vi "set temperature program.vi"(8 "Detectors":T2, 11 "Serial Port":refnum<visa-resource-name>) -> (0 "Canceled":bool, 1 "run time":dbl format="%<%H:%M:%S%0u>t", 2 "delta x":dbl=0.05 format="%.5f", 3 "Serial Port":refnum<visa-resource-name>, 4 "data points":u8)   [LabVIEW 2012]
uses:
  detector.ctl
panel:
  in  "data rate":T1(ring)
  in  "Inj B Temp":u16=100 max=400 step=1
  in  "cancel":bool
  out "Message":string
  out "response":string[](array[string])
  in  "Ramps":T3(ring)
  in  "Oven Equilibrium time":sgl=10.0 min=0 max=650 step=0.01 format="%.2f"
  in  "Oven Temperature":T4={"initial temp"=0, "initial time"=0.0, "rate"=10.0, "final temp"=0, "final time"=0.0, "rate A"=0.0, "final temp A"=0, "final time A"=1.4013e-43, "rate B"=10.0, "final temp B"=0, "final time B"=0.0} {"initial temp" min=-80 max=450 step=1; "final temp B" min=-80 max=450 step=1; "initial time" min=0 max=650 step=0.01 format="%.2f"; "final time B" min=0 max=650 step=0.01 format="%.2f"; "final temp A" min=-80 max=450 step=1; "rate B" min=0 max=70 step=0.1 format="%.1f"; "final time A" min=0 max=650 step=0.01 format="%.2f"; "final temp" min=-80 max=450 step=1; "rate A" min=0 max=70 step=0.1 format="%.1f"; "final time" min=0 max=650 step=0.01 format="%.2f"; "rate" min=0 max=70 step=0.1 format="%.1f"}
  in  "done":bool
  out "Temperatures":cluster{sgl[], u16[]}[](graph)
  in  "Det B temp":u16=100 max=400 step=1
  in  "Det A temp":u16=100 max=450 step=1
  in  "Inj A Temp":u16=100 max=400 step=1
  # "°C"
  # "Decimal minutes"
  # "Temperatures"
  # "times in decimal minutes\ntemperatures in °C"
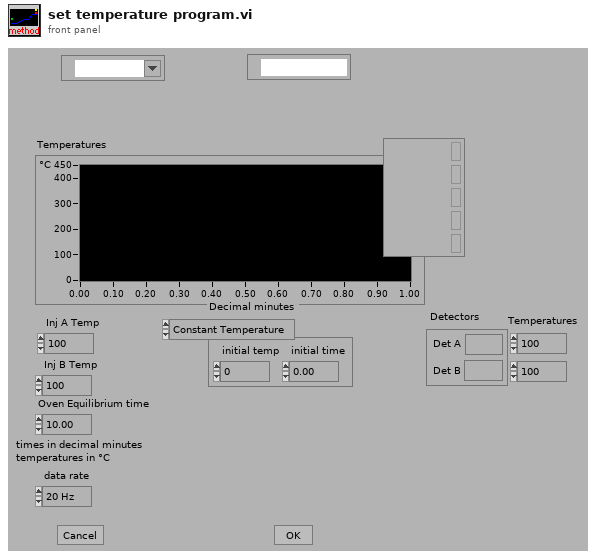
[diagram p1: front panel]
types:
  T1 = enum16{"20 Hz", "10 Hz", "5 Hz", "2.5 Hz", "1.25 Hz"}
  T2 = typedef "detector.ctl" = cluster{"Det A":string, "Det B":string}
  T3 = enum16{"Constant Temperature", "One Temperature Ramp", "Two Temperature Ramps", "Three Temperature Ramps"}
  T4 = cluster{"initial temp":i16, "initial time":sgl, "rate":sgl, "final temp":i16, "final time":sgl, "rate A":sgl, "final temp A":i16, "final time A":sgl, "rate B":sgl, "final temp B":i16, "final time B":sgl}
  T5 = cluster{"Version":sgl, "Initial Temp":sgl, "Oven On/Off":sgl, "Cryogenic  On/Off":sgl, "Oven Max":sgl, "Equib Time":sgl, "Initial Time":sgl, "Rate":dbl, "Final Temp":dbl, "Final Time":dbl, "Rate A":dbl, "Final Temp A":dbl, "Final Time A":dbl, "Rate B":dbl, "Final Temp B":dbl, "Final Time B":dbl, "Inj. A Temp":dbl, "Inj. A Temp On/Off":dbl, "Inj. B Temp":dbl, "Inj. B Temp On/Off":dbl, "Det. A Temp":dbl, "Det. A Temp On/Off":dbl, "Det. B Temp":dbl, "Det. B Temp On/Off":dbl, "Signal 1 Address":dbl, "Signal 1 Range":dbl, "Signal 1 Zero":dbl, "Signal 1 Zero On/Off":dbl, "Signal 1 Attn.":dbl, "Signal 1 Attn. On/Off":dbl, "Signal 2 Address":dbl, "Signal 2 Range":dbl, "Signal 2 Zero":dbl, "Signal 2 Zero On/Off":dbl, "Signal 2 Attn.":dbl, "Signal 2 Attn. On/Off":dbl, "Det. A On/Off":dbl, "Det. A Polarity":dbl, "Det. A Time":dbl, "Det. B On/Off":dbl, "Det. B Polarity":dbl, "Det. B Time":dbl, "Purge A On/Off":dbl, "Purge A On Time":dbl, "Purge A Off Time":dbl, "Purge B On/Off":dbl, "Purge B On Time":dbl, "Purge B Off Time":dbl}
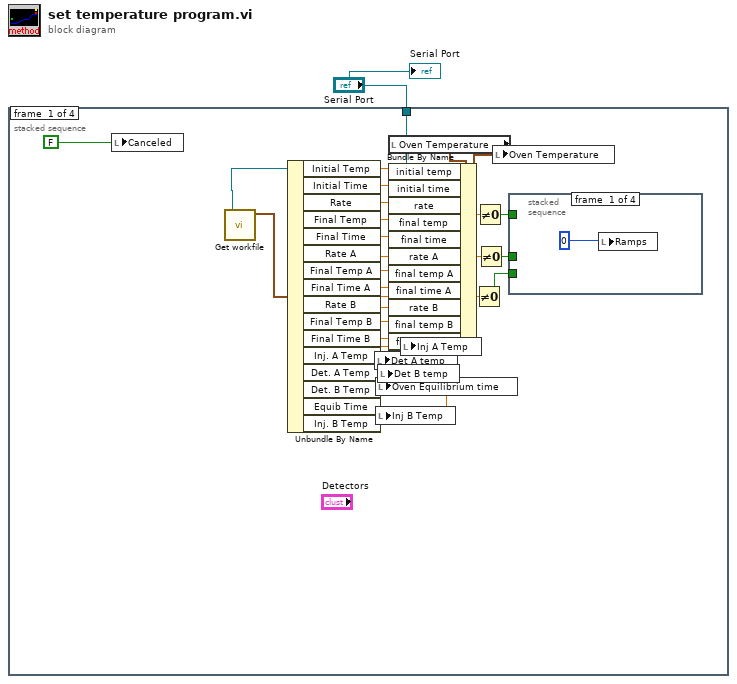
[diagram p0: block diagram]
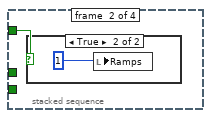
[diagram p2: hidden frame]
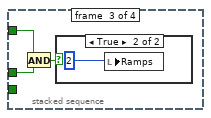
[diagram p4: hidden frame]
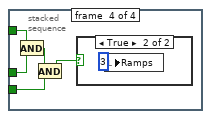
[diagram p6: hidden frame]
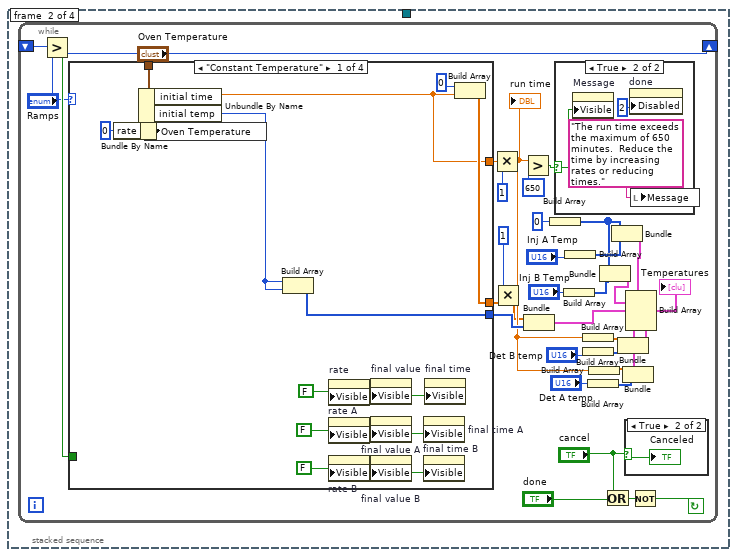
[diagram p8: hidden frame]
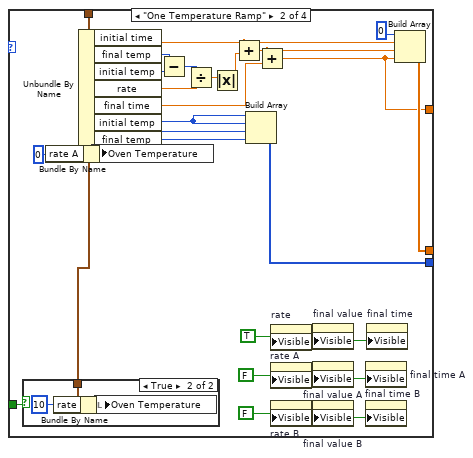
[diagram p10: hidden frame]
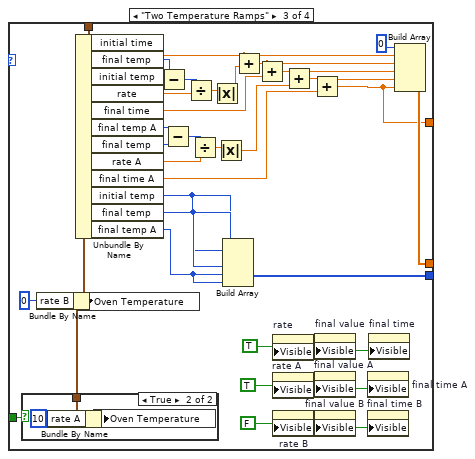
[diagram p12: hidden frame]
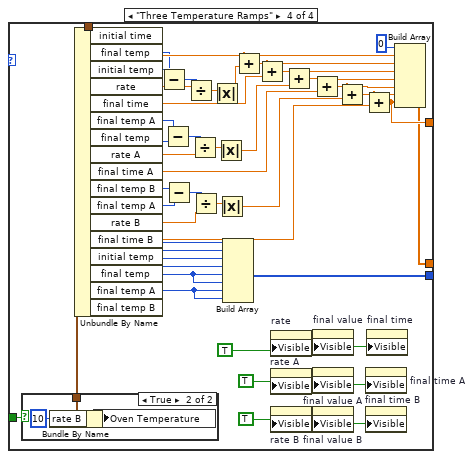
[diagram p14: hidden frame]
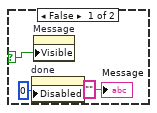
[diagram p16: hidden frame]
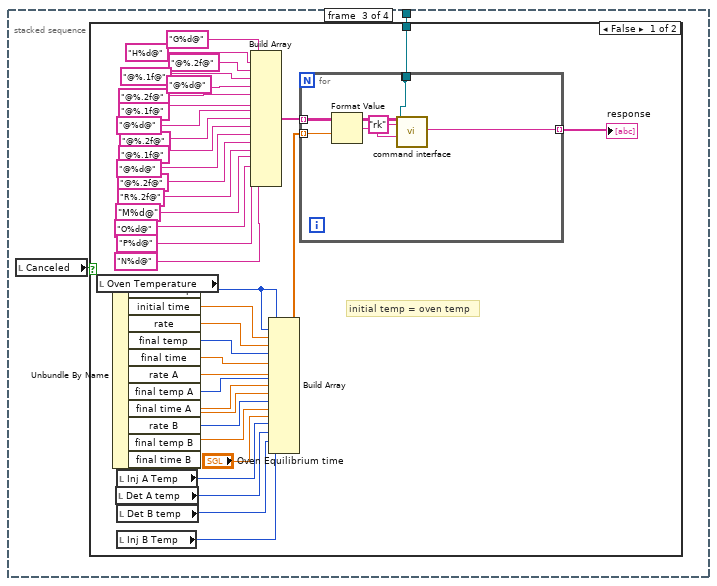
[diagram p17: hidden frame]
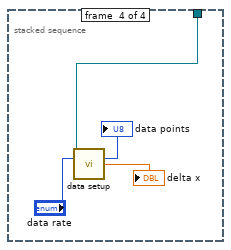
[diagram p19: hidden frame]
diagram:
  n1 = stacked-sequence {
    tunnel: "Serial Port" -> [w3 _ w195 w241]
    frame #0 {
      n2 = local write "Canceled"(FALSE) -> ()
      n3 = call "Get workfile.vi"("Serial Port"=w3) -> ("Workfile"=w24:T5)  [unwired: 4 in, 2 out]
      n4 = Unbundle By Name(w24) -> ("Initial Temp"=w22:sgl, "Initial Time"=w21:sgl, "Rate"=w20:dbl, "Final Temp"=w19:dbl, "Final Time"=w18:dbl, "Rate A"=w17:dbl, "Final Temp A"=w16:dbl, "Final Time A"=w15:dbl, "Rate B"=w14:dbl, "Final Temp B"=w13:dbl, "Final Time B"=w12:dbl, "Inj. A Temp"=w9:dbl, "Det. A Temp"=w10:dbl, "Det. B Temp"=w11:dbl, "Equib Time"=w8:sgl, "Inj. B Temp"=w2:dbl)
      n5 = local write "Det A temp"(w10) -> ()
      n6 = local write "Oven Equilibrium time"(w8) -> ()
      n7 = local write "Inj B Temp"(w2) -> ()
      n8 = local write "Det B temp"(w11) -> ()
      n9 = local read "Oven Temperature"() -> (w23:T4)
      n10 = Bundle By Name(cluster=w23, "initial temp"=w22, "initial time"=w21, "rate"=w20, "final temp"=w19, "final time"=w18, "rate A"=w17, "final temp A"=w16, "final time A"=w15, "rate B"=w14, "final temp B"=w13, "final time B"=w12) -> (w4:T4)
      n11 = local write "Inj A Temp"(w9) -> ()
      n12 = Not Equal To 0?(x=w14) -> (x != 0?=w5:bool)
      n13 = Not Equal To 0?(x=w20) -> (x != 0?=w7:bool)
      n14 = Not Equal To 0?(x=w17) -> (x != 0?=w6:bool)
      n15 = local write "Oven Temperature"(w4) -> ()
      n16 = stacked-sequence {
        tunnel: w7 -> [_ w27 w30 w37]
        tunnel: w6 -> [_ _ w29 w36]
        tunnel: w5 -> [_ _ _ w34]
        frame #0 {
          n17 = local write "Ramps"(0) -> ()
        }
        frame #1 {
          n18 = case shown="True" w27 {
            frame False {
            }
            frame True {
              n19 = local write "Ramps"(1) -> ()
            }
          }
        }
        frame #2 {
          n20 = And(x=w30, y=w29) -> (x .and. y?=w31:bool)
          n21 = case shown="True" w31 {
            frame False {
            }
            frame True {
              n22 = local write "Ramps"(2) -> ()
            }
          }
        }
        frame #3 {
          n23 = And(x=w37, y=w36) -> (x .and. y?=w35:bool)
          n24 = And(x=w35, y=w34) -> (x .and. y?=w33:bool)
          n25 = case shown="True" w33 {
            frame False {
            }
            frame True {
              n26 = local write "Ramps"(3) -> ()
            }
          }
        }
      }
    }
    frame #1 {
      n27 = while {
        shift-left: _ -> [w55]
        shift-right: ["Ramps"] -> _
        stop <- w73 continue-if-true
        n28 = Greater?(x="Ramps", y=w55) -> (0:w56:bool)
        n29 = case shown="\"Constant Temperature\"" "Ramps" {
          tunnel: [w78 w87 w112 w185] -> w44
          tunnel: [w85 w107 w142 w184] -> w50
          tunnel: [w84 w104 w138 w170] -> w47
          tunnel: "Oven Temperature" -> [w77 w93 w118 w150]
          tunnel: w56 -> [_ w86 w111 w147]
          frame "Constant Temperature" {
            w80 = FALSE
            w81 = FALSE
            w82 = FALSE
            n30 = Bundle By Name(cluster=w77, "rate"=0) -> (w76:T4)
            n31 = Unbundle By Name(w77) -> ("initial time"=w78:sgl, "initial temp"=w79:i16)
            n32 = local write "Oven Temperature"(w76) -> ()
            n33 = Build Array(w79, w79) -> (w85:i16[])
            n34 = property on="rate" class="DigNum (strict)"("Visible"=w82) -> ()  [unwired: 2 in, 2 out]
            n35 = property on="rate A" class="DigNum (strict)"("Visible"=w81) -> ()  [unwired: 2 in, 2 out]
            n36 = property on="rate B" class="DigNum (strict)"("Visible"=w80) -> ()  [unwired: 2 in, 2 out]
            n37 = property on="final value" class="DigNum (strict)"("Visible"=w82) -> ()  [unwired: 2 in, 2 out]
            n38 = property on="final value A" class="DigNum (strict)"("Visible"=w81) -> ()  [unwired: 2 in, 2 out]
            n39 = property on="final value B" class="DigNum (strict)"("Visible"=w80) -> ()  [unwired: 2 in, 2 out]
            n40 = property on="final time A" class="DigNum (strict)"("Visible"=w81) -> ()  [unwired: 2 in, 2 out]
            n41 = property on="final time B" class="DigNum (strict)"("Visible"=w80) -> ()  [unwired: 2 in, 2 out]
            n42 = property on="final time" class="DigNum (strict)"("Visible"=w82) -> ()  [unwired: 2 in, 2 out]
            n43 = Build Array(0, w78) -> (w84:sgl[])
          }
          frame "One Temperature Ramp" {
            w90 = FALSE
            w91 = FALSE
            w92 = TRUE
            n44 = case shown="True" w86 {
              tunnel: w93 -> [_ w108]
              frame False {
              }
              frame True {
                n45 = Bundle By Name(cluster=w108, "rate"=10) -> (w109:T4)
                n46 = local write "Oven Temperature"(w109) -> ()
              }
            }
            n47 = Bundle By Name(cluster=w93, "rate A"=0) -> (w89:T4)
            n48 = Unbundle By Name(w93) -> ("initial time"=w100:sgl, "final temp"=w94:i16, "initial temp"=w95:i16, "rate"=w97:sgl, "final time"=w103:sgl, "initial temp"=w105:i16, "final temp"=w106:i16)
            n49 = local write "Oven Temperature"(w89) -> ()
            n50 = Subtract(x=w94, y=w95) -> (x-y=w96:i16)
            n51 = Divide(x=w96, y=w97) -> (x/y=w98:sgl)
            n52 = Absolute Value(x=w98) -> (abs(x)=w101:sgl)
            n53 = Add(x=w100, y=w101) -> (x+y=w102:sgl)
            n54 = Build Array(w105, w105, w106, w106) -> (w107:i16[])
            n55 = Add(x=w102, y=w103) -> (x+y=w87:sgl)
            n56 = property on="rate" class="DigNum (strict)"("Visible"=w92) -> ()  [unwired: 2 in, 2 out]
            n57 = property on="rate A" class="DigNum (strict)"("Visible"=w91) -> ()  [unwired: 2 in, 2 out]
            n58 = property on="rate B" class="DigNum (strict)"("Visible"=w90) -> ()  [unwired: 2 in, 2 out]
            n59 = property on="final value" class="DigNum (strict)"("Visible"=w92) -> ()  [unwired: 2 in, 2 out]
            n60 = property on="final value A" class="DigNum (strict)"("Visible"=w91) -> ()  [unwired: 2 in, 2 out]
            n61 = property on="final value B" class="DigNum (strict)"("Visible"=w90) -> ()  [unwired: 2 in, 2 out]
            n62 = property on="final time A" class="DigNum (strict)"("Visible"=w91) -> ()  [unwired: 2 in, 2 out]
            n63 = property on="final time B" class="DigNum (strict)"("Visible"=w90) -> ()  [unwired: 2 in, 2 out]
            n64 = property on="final time" class="DigNum (strict)"("Visible"=w92) -> ()  [unwired: 2 in, 2 out]
            n65 = Build Array(0, w100, w102, w87) -> (w104:sgl[])
          }
          frame "Two Temperature Ramps" {
            w115 = FALSE
            w116 = TRUE
            w117 = TRUE
            n66 = case shown="True" w111 {
              tunnel: w118 -> [_ w143]
              frame False {
              }
              frame True {
                n67 = Bundle By Name(cluster=w143, "rate A"=10) -> (w144:T4)
                n68 = local write "Oven Temperature"(w144) -> ()
              }
            }
            n69 = Bundle By Name(cluster=w118, "rate B"=0) -> (w114:T4)
            n70 = Unbundle By Name(w118) -> ("initial time"=w130:sgl, "final temp"=w119:i16, "initial temp"=w120:i16, "rate"=w122:sgl, "final time"=w133:sgl, "final temp A"=w126:i16, "final temp"=w127:i16, "rate A"=w128:sgl, "final time A"=w137:sgl, "initial temp"=w139:i16, "final temp"=w140:i16, "final temp A"=w141:i16)
            n71 = local write "Oven Temperature"(w114) -> ()
            n72 = Subtract(x=w119, y=w120) -> (x-y=w121:i16)
            n73 = Subtract(x=w126, y=w127) -> (x-y=w125:i16)
            n74 = Divide(x=w121, y=w122) -> (x/y=w123:sgl)
            n75 = Divide(x=w125, y=w128) -> (x/y=w124:sgl)
            n76 = Absolute Value(x=w123) -> (abs(x)=w131:sgl)
            n77 = Absolute Value(x=w124) -> (abs(x)=w135:sgl)
            n78 = Build Array(w139, w139, w140, w140, w141, w141) -> (w142:i16[])
            n79 = Add(x=w130, y=w131) -> (x+y=w132:sgl)
            n80 = Add(x=w132, y=w133) -> (x+y=w134:sgl)
            n81 = property on="rate" class="DigNum (strict)"("Visible"=w117) -> ()  [unwired: 2 in, 2 out]
            n82 = property on="rate A" class="DigNum (strict)"("Visible"=w116) -> ()  [unwired: 2 in, 2 out]
            n83 = property on="rate B" class="DigNum (strict)"("Visible"=w115) -> ()  [unwired: 2 in, 2 out]
            n84 = Add(x=w134, y=w135) -> (x+y=w136:sgl)
            n85 = Add(x=w136, y=w137) -> (x+y=w112:sgl)
            n86 = property on="final value" class="DigNum (strict)"("Visible"=w117) -> ()  [unwired: 2 in, 2 out]
            n87 = property on="final value A" class="DigNum (strict)"("Visible"=w116) -> ()  [unwired: 2 in, 2 out]
            n88 = property on="final value B" class="DigNum (strict)"("Visible"=w115) -> ()  [unwired: 2 in, 2 out]
            n89 = property on="final time A" class="DigNum (strict)"("Visible"=w116) -> ()  [unwired: 2 in, 2 out]
            n90 = property on="final time B" class="DigNum (strict)"("Visible"=w115) -> ()  [unwired: 2 in, 2 out]
            n91 = property on="final time" class="DigNum (strict)"("Visible"=w117) -> ()  [unwired: 2 in, 2 out]
            n92 = Build Array(0, w130, w132, w134, w136, w112) -> (w138:sgl[])
          }
          frame "Three Temperature Ramps" {
            w146 = TRUE
            w148 = TRUE
            w149 = TRUE
            n93 = case shown="True" w147 {
              tunnel: w150 -> [_ w186]
              frame False {
              }
              frame True {
                n94 = Bundle By Name(cluster=w186, "rate B"=10) -> (w187:T4)
                n95 = local write "Oven Temperature"(w187) -> ()
              }
            }
            n96 = Unbundle By Name(w150) -> ("initial time"=w162:sgl, "final temp"=w151:i16, "initial temp"=w152:i16, "rate"=w154:sgl, "final time"=w165:sgl, "final temp A"=w158:i16, "final temp"=w159:i16, "rate A"=w160:sgl, "final time A"=w169:sgl, "final temp B"=w173:i16, "final temp A"=w174:i16, "rate B"=w175:sgl, "final time B"=w178:sgl, "initial temp"=w180:i16, "final temp"=w181:i16, "final temp A"=w182:i16, "final temp B"=w183:i16)
            n97 = Subtract(x=w151, y=w152) -> (x-y=w153:i16)
            n98 = Subtract(x=w158, y=w159) -> (x-y=w157:i16)
            n99 = Subtract(x=w173, y=w174) -> (x-y=w171:i16)
            n100 = Divide(x=w153, y=w154) -> (x/y=w155:sgl)
            n101 = Divide(x=w157, y=w160) -> (x/y=w156:sgl)
            n102 = Divide(x=w171, y=w175) -> (x/y=w172:sgl)
            n103 = Absolute Value(x=w155) -> (abs(x)=w163:sgl)
            n104 = Absolute Value(x=w156) -> (abs(x)=w167:sgl)
            n105 = Absolute Value(x=w172) -> (abs(x)=w176:sgl)
            n106 = Build Array(w180, w180, w181, w181, w182, w182, w183, w183) -> (w184:i16[])
            n107 = Add(x=w162, y=w163) -> (x+y=w164:sgl)
            n108 = Add(x=w164, y=w165) -> (x+y=w166:sgl)
            n109 = property on="rate" class="DigNum (strict)"("Visible"=w146) -> ()  [unwired: 2 in, 2 out]
            n110 = property on="rate A" class="DigNum (strict)"("Visible"=w149) -> ()  [unwired: 2 in, 2 out]
            n111 = property on="rate B" class="DigNum (strict)"("Visible"=w148) -> ()  [unwired: 2 in, 2 out]
            n112 = Add(x=w166, y=w167) -> (x+y=w168:sgl)
            n113 = Add(x=w168, y=w169) -> (x+y=w177:sgl)
            n114 = property on="final value" class="DigNum (strict)"("Visible"=w146) -> ()  [unwired: 2 in, 2 out]
            n115 = property on="final value A" class="DigNum (strict)"("Visible"=w149) -> ()  [unwired: 2 in, 2 out]
            n116 = property on="final value B" class="DigNum (strict)"("Visible"=w148) -> ()  [unwired: 2 in, 2 out]
            n117 = Add(x=w177, y=w176) -> (x+y=w179:sgl)
            n118 = Add(x=w179, y=w178) -> (x+y=w185:sgl)
            n119 = property on="final time A" class="DigNum (strict)"("Visible"=w149) -> ()  [unwired: 2 in, 2 out]
            n120 = property on="final time B" class="DigNum (strict)"("Visible"=w148) -> ()  [unwired: 2 in, 2 out]
            n121 = property on="final time" class="DigNum (strict)"("Visible"=w146) -> ()  [unwired: 2 in, 2 out]
            n122 = Build Array(0, w162, w164, w166, w168, w177, w179, w185) -> (w170:sgl[])
          }
        }
        n123 = Multiply(x=w44, y=1) -> (x*y=w49:sgl)
        "run time" <- w49
        n124 = Multiply(x=1, y=w47) -> (x*y=w45:sgl[])
        n125 = Greater?(x=w49, y=650) -> (0:w71:bool)
        n126 = Bundle(w45, w50) -> (w69:cluster{sgl[], i16[]})  [unwired: 1 in]
        n127 = Build Array(i16 0) -> (w40:i16[])
        n128 = case shown="True" w71 {
          selector: w71 -> [w189 w192]
          frame False {
            n129 = property on="done" class="Bool"("Disabled"=0) -> ()  [unwired: 2 in, 2 out]
            n130 = property on="Message" class="Str"("Visible"=w189) -> ()  [unwired: 2 in, 2 out]
            "Message" <- ""
          }
          frame True {
            n131 = property on="Message" class="Str"("Visible"=w192) -> ()  [unwired: 2 in, 2 out]
            n132 = property on="done" class="Bool"("Disabled"=2) -> ()  [unwired: 2 in, 2 out]
            n133 = local write "Message"("The run time exceeds the maximum of 650 minutes.  Reduce the time by increasing rates or reducing times.") -> ()
          }
        }
        n134 = Build Array("Inj B Temp") -> (w41:u16[])
        n135 = Build Array("Inj A Temp") -> (w66:u16[])
        n136 = Build Array(w49) -> (w63:sgl[])
        n137 = Build Array("Det B temp") -> (w62:u16[])
        n138 = Build Array("Det A temp") -> (w60:u16[])
        n139 = Build Array(w49) -> (w61:sgl[])
        n140 = Bundle(w40, w41) -> (w39:cluster{i16[], u16[]})  [unwired: 1 in]
        n141 = Or(x="cancel", y="done") -> (x .or. y?=w52:bool)
        n142 = Bundle(w40, w66) -> (w43:cluster{i16[], u16[]})  [unwired: 1 in]
        n143 = Bundle(w63, w62) -> (w59:cluster{sgl[], u16[]})  [unwired: 1 in]
        n144 = Bundle(w61, w60) -> (w58:cluster{sgl[], u16[]})  [unwired: 1 in]
        n145 = case shown="True" "cancel" {
          selector: "cancel" -> [_ w74]
          frame False {
          }
          frame True {
            "Canceled" <- w74
          }
        }
        n146 = Build Array(w43, w39, w69, w59, w58) -> (→"Temperatures":cluster{sgl[], u16[]}[])
        n147 = Not(x=w52) -> (.not. x?=w73:bool)
      }
    }
    frame #2 {
      n148 = local read "Canceled"() -> (w196:bool)
      n149 = case shown="False" w196 {
        tunnel: w195 -> [w201 _]
        frame False {
          # "initial temp = oven temp"
          n150 = local read "Oven Temperature"() -> (w203:T4)
          n151 = Unbundle By Name(w203) -> ("initial temp"=w198:i16, "initial time"=w204:sgl, "rate"=w205:sgl, "final temp"=w206:i16, "final time"=w208:sgl, "rate A"=w209:sgl, "final temp A"=w207:i16, "final time A"=w210:sgl, "rate B"=w211:sgl, "final temp B"=w212:i16, "final time B"=w213:sgl)
          n152 = local read "Det A temp"() -> (w229:u16)
          n153 = local read "Inj A Temp"() -> (w228:u16)
          n154 = local read "Det B temp"() -> (w230:u16)
          n155 = local read "Inj B Temp"() -> (w200:u16)
          n156 = Build Array("G%d@", "H%d@", "@%.2f@", "@%.1f@", "@%d@", "@%.2f@", "@%.1f@", "@%d@", "@%.2f@", "@%.1f@", "@%d@", "@%.2f@", "R%.2f@", "M%d@", "O%d@", "P%d@", "N%d@") -> (w227:string[])
          n157 = Build Array(w198, w198, w204, w205, w206, w208, w209, w207, w210, w211, w212, w213, "Oven Equilibrium time", w228, w229, w230, w200) -> (w202:sgl[])
          n158 = for {
            tunnel: w227 -> [w240] mode=indexing
            tunnel: w202 -> [w239] mode=indexing
            tunnel: [w235] -> _ mode=indexing
            tunnel: [w236] -> w234 mode=indexing
            tunnel: w201 -> [w235]
            n159 = Format Value(format string=w240, value (0)=w239) -> (output string=w238:string)  [unwired: 1 in]
            n160 = call "command interface.vi"("Parameter"=w238, "command"="rk", "Serial Port"=w235) -> ("response"=w236:string)  [unwired: 4 in, 3 out]
          }
          "response" <- w234
        }
        frame True {
        }
      }
    }
    frame #3 {
      n161 = call "data setup.vi"("Serial Port"=w241, "data rate"="data rate") -> ("data points"=→"data points":u8, "delta x"=→"delta x":dbl)  [unwired: 11 in, 1 out]
    }
  }
  "Serial Port" <- "Serial Port"
